vi "Write Scale Range Minor Increment.vi"(6 "Control Ref Queue":T1, 8 "error in (no error)":errorcluster, 9 "Index":i32, 10 "Minor Increment":dbl, 11 "2D Plot.lvclass in":refnum<class "2D Plot.lvclass">) -> (0 "error out":errorcluster, 3 "2D Plot.lvclass out":refnum<class "2D Plot.lvclass">)   [LabVIEW 2020, in "2D Plot.lvclass"]
uses:
  <vilib>/Math Plots/2D Math Plots/2D Plot/2D Plot/2D Plot.lvclass
  <vilib>/Math Plots/2D Math Plots/2D Plot/Action String/2DMathPlot Ctrl Act Queue.ctl
  <vilib>/Math Plots/2D Math Plots/2D Plot/Action String/2DMathPlot Ctrl Act Cluster.ctl
  <vilib>/Math Plots/2D Math Plots/2D Plot/Action String/2DMathPlot State Class.ctl
  <vilib>/Math Plots/2D Math Plots/2D Plot/2D Plot/2D Plot.lvclass/2D Plot.ctl
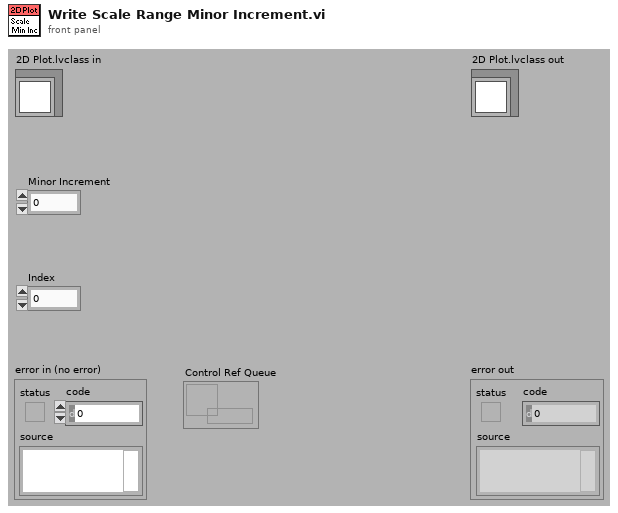
[diagram p1: front panel]
types:
  T1 = typedef "2DMathPlot Ctrl Act Queue.ctl" = refnum<queue>
  T2 = typedef "2D Plot.lvclass/Scale Array.ctl" = T3[]
  T3 = typedef "2D Plot.lvclass/Scale Cluster.ctl" = cluster{"General":cluster{"Editable":bool, "Flipped":bool, "Mapping Mode":u8, "Visible":bool, "Style":u8, "Scale Fit":u8}, "Offset and Multiplier":T4, "Range":cluster{"Minimum":dbl, "Maximum":dbl, "Increment":dbl, "Minor Increment":dbl, "Start":dbl}, "Tick Color":cluster{"Major Color":u32, "Minor Color":u32}, "Gird Color":cluster{"Major Color":u32, "Minor Color":u32}, "Marker":cluster{"Visible":bool, "FG Color":u32, "BG Color":u32, "Font Name":string, "Font Size":u32, "Font Bold":bool, "Font Italic":bool, "Font Strikeout":bool, "Font Underline":bool}, "Name Label":cluster{"Visible":bool, "FG Color":u32, "BG Color":u32, "Font Name":string, "Font Size":u32, "Font Bold":bool, "Font Italic":bool, "Font Strikeout":bool, "Font Underline":bool, "Justification":enum16{"Left", "Center", "Right"}, "Text":string}}
  T4 = typedef "LVOffsetAndMultiplierTypeDef.ctl" = cluster{"Offset":dbl, "Multiplier":dbl}
  T5 = typedef "2DMathPlot Ctrl Act Cluster.ctl" = cluster{"Plot Area Ref":refnum<vi>, "Z Axis Ref":refnum<vi>, "Legend Ref":refnum<vi>, "XControl Ref":refnum<vi>, "Facade Ref":refnum<vi>, "Display State Change Class":T6}
  T6 = typedef "2DMathPlot State Class.ctl" = enum16{"Update All (Undo)", "Update General", "Update Appearance", "Update Format", "Update Scale", "Update Marker", "Update Cursor", "None"}
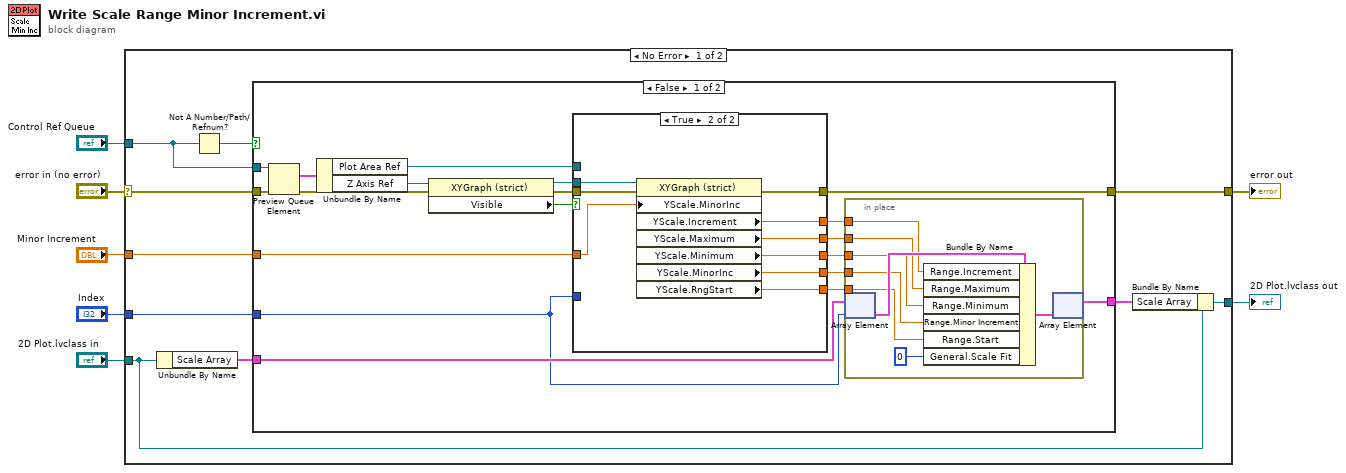
[diagram p0: block diagram]
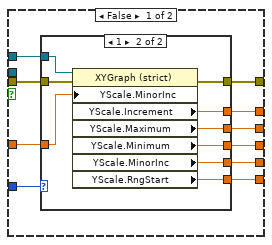
[diagram p2: hidden frame]
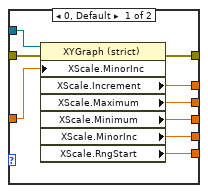
[diagram p3: hidden frame]
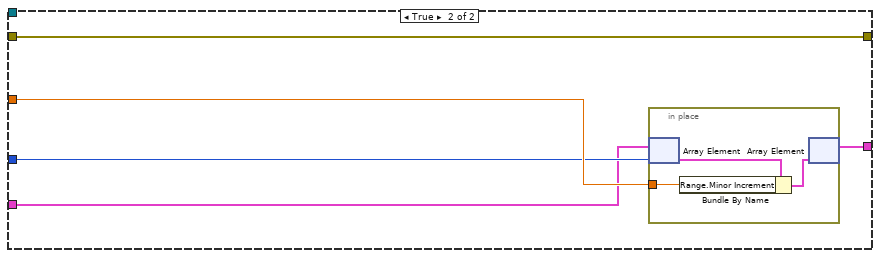
[diagram p4: hidden frame]
diagram:
  n1 = case shown="No Error" "error in (no error)" {
    selector: "error in (no error)" -> [w11 w91]
    tunnel: "2D Plot.lvclass in" -> [w17 w90]
    tunnel: [w16 w90] -> w2
    tunnel: "Control Ref Queue" -> [w9 _]
    tunnel: [w13 w91] -> w1
    tunnel: "Index" -> [w12 _]
    tunnel: "Minor Increment" -> [w10 _]
    frame No Error {
      n2 = Unbundle By Name(w17) -> ("Scale Array"=w15:T2)
      n3 = Not A Number/Path/Refnum?(number/path/refnum=w9) -> (NaN/Path/Refnum?=w8:bool)
      n4 = case shown="False" w8 {
        tunnel: w9 -> [w36 _]
        tunnel: w15 -> [w29 w84]
        tunnel: [w28 w83] -> w14
        tunnel: [w27 w82] -> w13
        tunnel: w12 -> [w21 w85]
        tunnel: w11 -> [w20 w82]
        tunnel: w10 -> [w19 w86]
        frame False {
          n5 = Preview Queue Element(queue=w36, error in (no error)=w20) -> (element=w35:T5, error out=w33:errorcluster)  [unwired: 1 in, 2 out]
          n6 = Unbundle By Name(w35) -> ("Plot Area Ref"=w32:refnum<vi>, "Z Axis Ref"=w18:refnum<vi>)
          n7 = property class="XYGraph (strict)"(reference=w18, error in=w33) -> (reference out=w31:refnum<vi>, error out=w30:errorcluster, "Visible"=w34:bool)
          n8 = case shown="True" w34 {
            tunnel: w30 -> [w54 w80]
            tunnel: [w53 w79] -> w27
            tunnel: w32 -> [w52 _]
            tunnel: w31 -> [_ w81]
            tunnel: w19 -> [w51 w78]
            tunnel: [w50 w77] -> w26
            tunnel: [w49 w76] -> w25
            tunnel: [w48 w75] -> w24
            tunnel: [w47 w74] -> w23
            tunnel: [w46 w73] -> w22
            tunnel: w21 -> [w45 _]
            frame False {
              n9 = case shown="1" w45 {
                tunnel: w54 -> [w62 w70]
                tunnel: [w61 w69] -> w53
                tunnel: w52 -> [w63 w71]
                tunnel: w51 -> [w60 w72]
                tunnel: [w59 w68] -> w50
                tunnel: [w58 w67] -> w49
                tunnel: [w57 w66] -> w48
                tunnel: [w56 w65] -> w47
                tunnel: [w55 w64] -> w46
                frame 0, Default {
                  n10 = property class="XYGraph (strict)"(reference=w63, error in=w62, "XScale.MinorInc"=w60) -> (error out=w61:errorcluster, "XScale.Increment"=w59:dbl, "XScale.Maximum"=w58:dbl, "XScale.Minimum"=w57:dbl, "XScale.MinorInc"=w56:dbl, "XScale.RngStart"=w55:dbl)  [unwired: 1 out]
                }
                frame 1 {
                  n11 = property class="XYGraph (strict)"(reference=w71, error in=w70, "YScale.MinorInc"=w72) -> (error out=w69:errorcluster, "YScale.Increment"=w68:dbl, "YScale.Maximum"=w67:dbl, "YScale.Minimum"=w66:dbl, "YScale.MinorInc"=w65:dbl, "YScale.RngStart"=w64:dbl)  [unwired: 1 out]
                }
              }
            }
            frame True {
              n12 = property class="XYGraph (strict)"(reference=w81, error in=w80, "YScale.MinorInc"=w78) -> (error out=w79:errorcluster, "YScale.Increment"=w77:dbl, "YScale.Maximum"=w76:dbl, "YScale.Minimum"=w75:dbl, "YScale.MinorInc"=w74:dbl, "YScale.RngStart"=w73:dbl)  [unwired: 1 out]
            }
          }
          n13 = in-place {
            in-place-border: w26 -> [w42]
            in-place-border: w25 -> [w41]
            in-place-border: w24 -> [w40]
            in-place-border: w23 -> [w39]
            in-place-border: w22 -> [w38]
            n14 = in-place-array #1(w29, w21) -> (w44:T3)
            n15 = Bundle By Name(cluster=w44, "Range.Increment"=w42, "Range.Maximum"=w41, "Range.Minimum"=w40, "Range.Minor Increment"=w39, "Range.Start"=w38, "General.Scale Fit"=u8 0) -> (w43:T3)
            n16 = in-place-array #1(w43) -> (w28:T2)  [unwired: 1 out]
          }
        }
        frame True {
          n17 = in-place {
            in-place-border: w86 -> [w87]
            n18 = in-place-array #2(w84, w85) -> (w89:T3)
            n19 = Bundle By Name(cluster=w89, "Range.Minor Increment"=w87) -> (w88:T3)
            n20 = in-place-array #2(w88) -> (w83:T2)  [unwired: 1 out]
          }
        }
      }
      n21 = Bundle By Name(cluster=w17, "Scale Array"=w14) -> (w16:refnum<class "2D Plot.lvclass">)
    }
    frame Error {
    }
  }
  "error out" <- w1
  "2D Plot.lvclass out" <- w2
